vi "CleanUp.vi"(8 "Error In":errorcluster, 11 "object in":refnum<class "Configuration.lvclass">) -> (0 "Error Out":errorcluster, 3 "object out":refnum<class "Configuration.lvclass">)   [LabVIEW 2023, in "HAL.lvlib" / "PXIe-5172.lvlib" / "Configuration.lvclass"]
uses:
  Configuration.lvclass
  Configuration.lvclass/Configuration.ctl
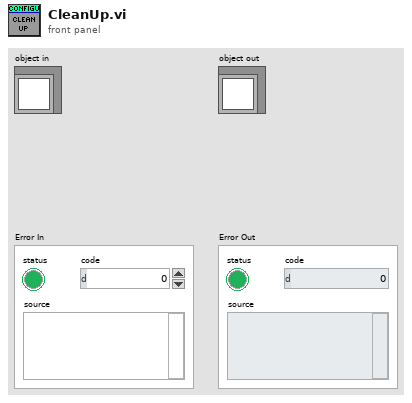
[diagram p1: front panel]
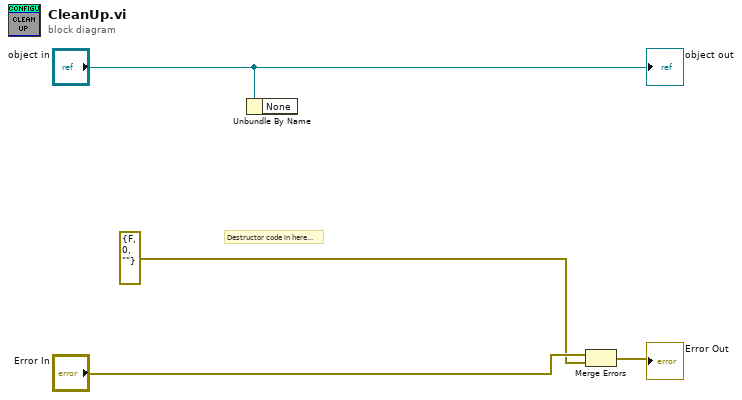
[diagram p0: block diagram]
diagram:
  # "Destructor code in here..."
  n1 = Unbundle By Name("object in") -> ()  [unwired: 1 out]
  n2 = Merge Errors("Error In", errorcluster {"status"=FALSE, "code"=0, "source"=""} ("error in (no error)")) -> (→"Error Out":errorcluster)
  "object out" <- "object in"
